vi "Dashboard Main.vi"() -> ()   [LabVIEW 2013]
uses:
  <vilib>/event_ctls.llb/eventvkey.ctl
  <vilib>/Rock Robotics/WPI/Dashboard/WPI_DashboardLogging Global.vi
  <vilib>/Utility/config.llb/Write Key (String).vi
  <vilib>/Utility/config.llb/Write Key (I32).vi
  <vilib>/Utility/config.llb/NI_LVConfig.lvlib
panel:
  out "Image Message":string="Timeout in Camera Communications"
  in  "Rec Mode":enum32{"Stop", "Record", "Playback"}(radio)
  in  "Dashboard Tab":T1(tab)
  out "RightJoystick":dbl(slide) scale=-1.0..1.0
  out "LeftJoystick":dbl(slide) scale=-1.0..1.0
  out "RightMotor":dbl(slide) scale=-1.0..1.0 scale format="%#.6g"
  out "StraightDrive":bool
  out "HalfDrive":bool
  in  "AccelRate":dbl(slide)=0.75 min=0.0 max=1.0 step=0.01 scale=0.0..1.0 scale format="%#_2g"
  out "LeftMotor":dbl(slide) scale=-1.0..1.0
  in  "Camera Settings":T2={"Frame Rate"=30, "Compression"=30, "Size"=1} {"Frame Rate" scale=1.0..30.0; "Size" items=["640x480", "320x240", "160x120"]}
  out "MotorSliders R":cluster{"MotorSlide1":dbl, "MotorSlide2":dbl} {"MotorSlide2" scale=-1.0..1.0 scale format="%#_2e"; "MotorSlide1" scale=-1.0..1.0 scale format="%#_2e"}
  out "MotorChart R":cluster{"Numeric":dbl, "Numeric":dbl}(graph)
  out "MotorSliders L":T3 {"MotorSlide4 2" scale=0.0..14.0 scale format="%#_2e"; "MotorSlide2" scale=-1.0..1.0 scale format="%#_2e"; "MotorSlide1" scale=-1.0..1.0 scale format="%#_2e"}
  out "MotorChart L":T4(graph)
  out "Mode":T5(ring)=enum."Auto Disabled"
  out "Camera IP":string
  in  "DB Camera Config":bool
  out "fps":dbl format="%#.1g"
  out "Mbps":dbl format="%#.1g"
  out "Mbps 2":bool
  out "LED 1":bool
  in  "Slider 1":dbl(slide) scale=0.0..100.0
  in  "Checkbox 2":bool
  in  "Checkbox 1":bool
  in  "Test Slider":dbl(slide) scale=0.0..100.0 scale format="%#_3g"
  in  "On/Off":bool caption="Solenoid"
  in  "Test Name":u16(ring) items=["Select the test to run...", "Example Test", "-------------------------------", "List of tests is built in robot code.", "Replace with your own automated tests."]
  in  "Test Tree":string(tree)
  in  "Motor":cluster{"Value":dbl, "Enable":bool} {"Value" scale=-1.0..1.0 scale format="%#_3g"}
  out "Progress":T6 {"Test Progress" scale=0.0..100.0}
  in  "Rev/Fwd":cluster{"Forward":bool, "Reverse":bool}
  in  "Test Ring":u16(ring) items=["Auto", "Fixed indoor", "Fixed outdoor 1", "Fixed outdoor 2", "Fixed fluorescent 1", "Fixed fluorescent 2", "Hold current"]
  in  "Listbox":i32(listbox)
  out "Tree":string(tree)
  out "Camera Image":T7(plugin-control)
  in  "Enable":bool
  # "Left"
  # "Front"
  # "Right"
  # "Battery"
  # "Customize by placing controls and indicators here and name to\nmatch Dashboard Variables on robot."
  # "This tab is a great place for autonomous settings and validation.\nCustomize by placing controls and indicators here and name to\nmatch Dashboard Variables on robot."
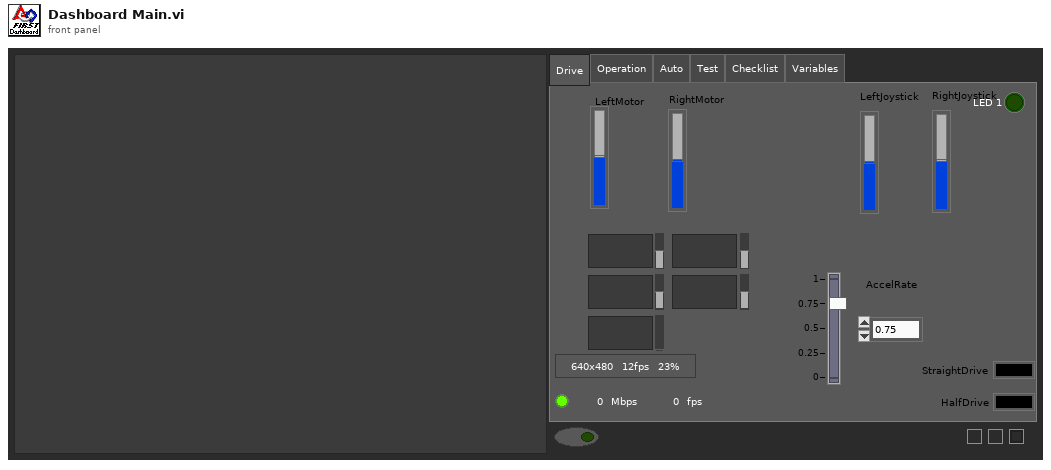
[diagram p1: front panel]
types:
  T1 = enum32{"Drive", "Operation", "Auto", "Test", "Checklist", "Variables"}
  T2 = cluster{"Frame Rate":i32, "Compression":i32, "Size":u16}
  T3 = cluster{"MotorSlide1":dbl, "MotorSlide2":dbl, "MotorSlide4 2":dbl}
  T4 = cluster{"Numeric":dbl, "Numeric":dbl, "Battery":sgl}
  T5 = enum8{"Tele-Op Disabled", "Tele-Op Enabled", "Auto Disabled", "Auto Enabled", "Test Disabled", "Test Enabled", ""}
  T6 = cluster{"Test Progress":u8, "Test Progress Text":string}
  T7 = typedef "IMAQ Image.ctl" = refnum<image>
  T8 = typedef "Image Type" = u32
  T9 = cluster{"Digital Inputs":bool[], "Digital Outputs":bool[]}
  T10 = cluster{"Competition mode":bool, "Robot Link":bool, "Autonomous":bool, "Enabled":bool, "E-Stop":bool, "Simulated":bool, "TestMode":bool, "Docked Window":bool}
  T11 = typedef "NI_LVConfig.lvlib/Config Data RefNum.ctl" = refnum<k1>
  T12 = typedef "eventvkey.ctl" = enum16{"ASCII", "Enter", "Return", "Shift", "Ctrl", "Alt", "Cmd", "Opt", "Caps", "NumLock", "Clear", "Break", "Up", "Down", "Left", "Right", "Insert", "Delete", "Home", "End", "PageUp", "PageDown", "Escape", "Help", "Pause", "ScrollLock", "F1", "F2", "F3", "F4", "F5", "F6", "F7", "F8", "F9", "F10", "F11", "F12", "F13", "F14", "F15", "F16", "F17", "F18", "F19", "F20", "F21", "F22", "F23", "F24", "Play", "VolumeUp", "VolumeDown", "Mute", "Two Byte Char"}
  T13 = cluster{"Image Size":bool, "Image Type":bool, "Pixel Value":bool, "ROI Information":bool, "Zoom Factor":bool}
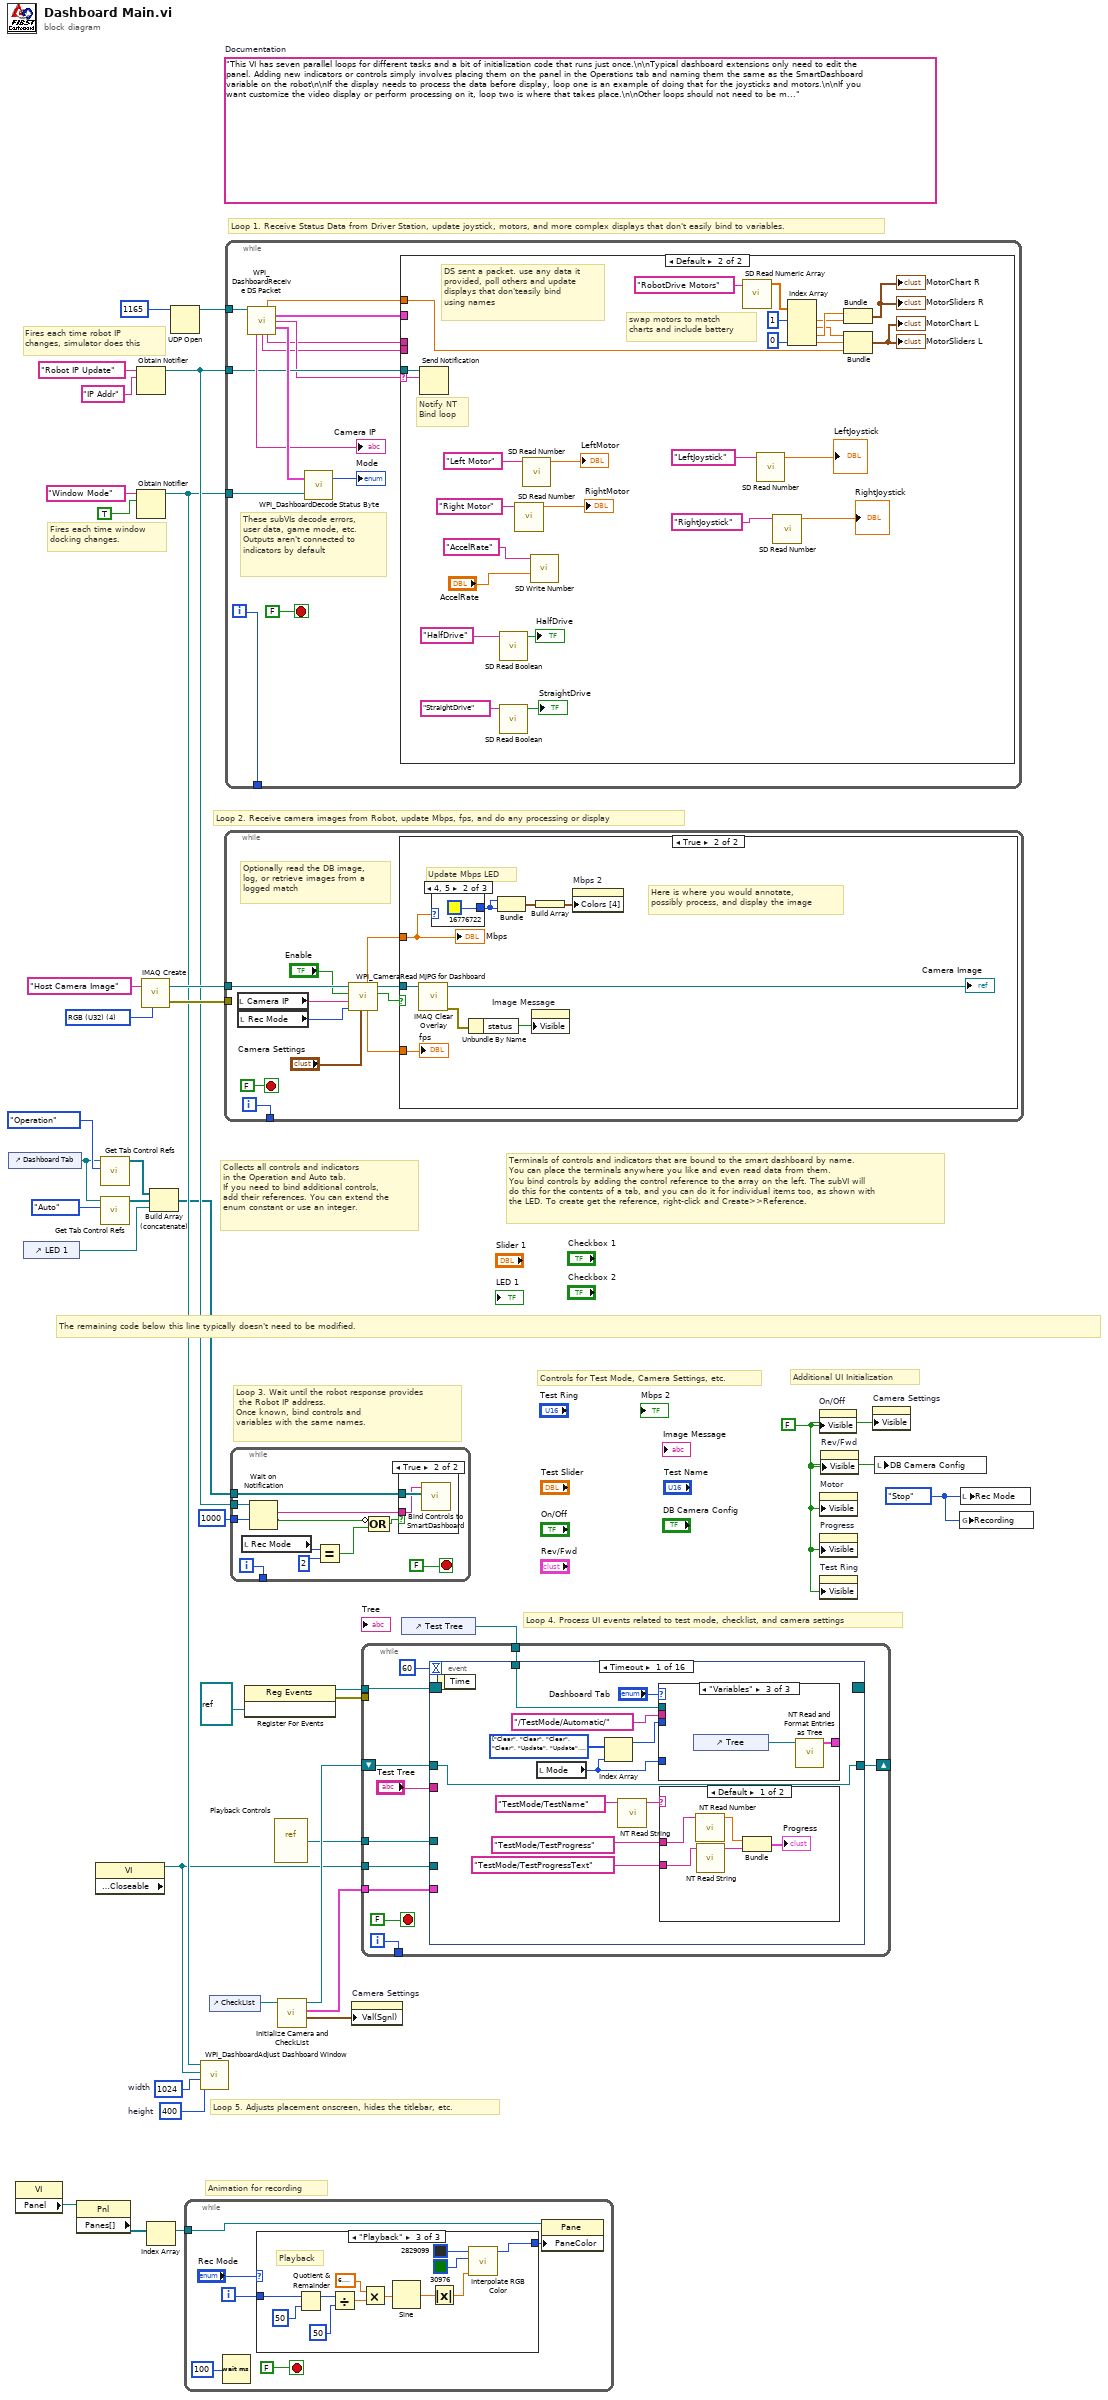
[diagram p0: block diagram]
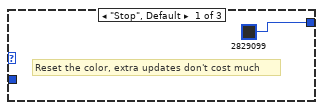
[diagram p2: hidden frame]
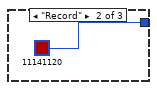
[diagram p3: hidden frame]
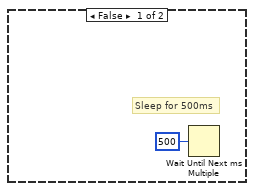
[diagram p5: hidden frame]
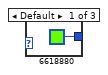
[diagram p6: hidden frame]
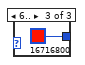
[diagram p7: hidden frame]
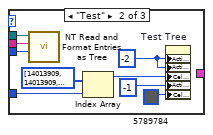
[diagram p9: hidden frame]
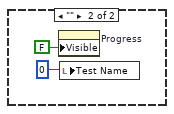
[diagram p10: hidden frame]
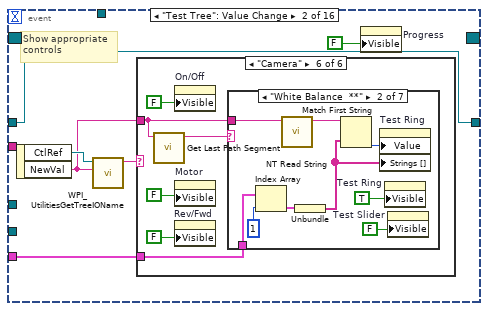
[diagram p11: hidden frame]
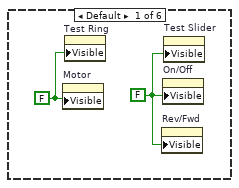
[diagram p12: hidden frame]
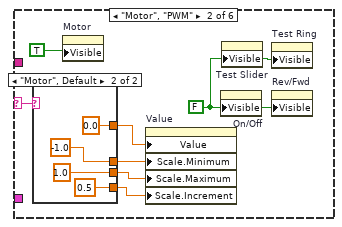
[diagram p13: hidden frame]
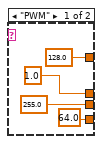
[diagram p14: hidden frame]
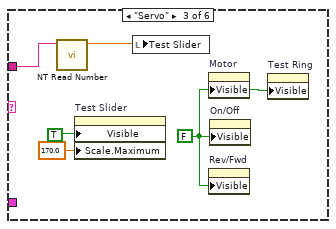
[diagram p15: hidden frame]
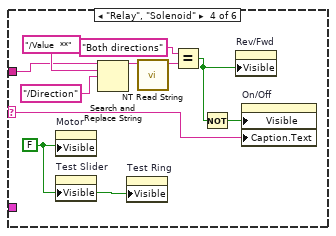
[diagram p16: hidden frame]
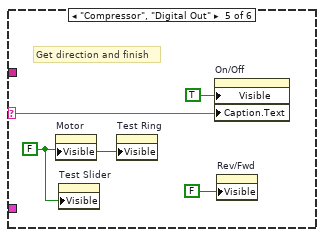
[diagram p17: hidden frame]
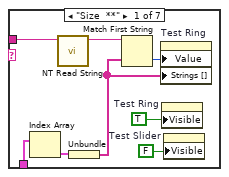
[diagram p18: hidden frame]
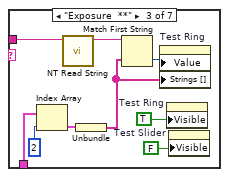
[diagram p19: hidden frame]
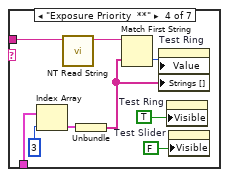
[diagram p20: hidden frame]
diagram:
  w8 = enum32{"Stop", "Record", "Playback"}."Stop" ("Rec Mode")
  w11 = 400  # height
  w12 = 1024  # width
  w25 = FALSE ("Visible")
  (unwired) "This VI has seven parallel loops for different tasks and a bit of initialization code that runs just once.\n\nTypical dashboard extensions only need to edit the panel. Adding new indicators or controls simply involves placing them on the panel in the Operations tab and naming them the same as the SmartDashboard variable on the robot\n\nIf the display needs to process the data before display, loop one is an example of doing that for the joysticks and motors.\n\nIf you want customize the video display or perform processing on it, loop two is where that takes place.\n\nOther loops should not need to be modified. They are pretty standard, and document the task they perform."  # Documentation
  w35 = T8 4 items=["Grayscale (U8)", "Grayscale (I16)", "Grayscale (SGL)", "Complex (CSG)", "RGB (U32)", "HSL (U32)", "RGB (U64)"] ("Image Type")
  # "Controls for Test Mode, Camera Settings, etc."
  # "Additional UI Initialization"
  # "Animation for recording"
  # "Fires each time robot IP\nchanges, simulator does this"
  # "Fires each time window\ndocking changes."
  # "Collects all controls and indicators\nin the Operation and Auto tab.\nIf you need to bind additional controls,\nadd their references. You can extend the\nenum constant or use an integer."
  # "The remaining code below this line typically doesn't need to be modified."
  # "Loop 4. Process UI events related to test mode, checklist, and camera settings"
  # "Terminals of controls and indicators that are bound to the smart dashboard by name.\nYou can place the terminals anywhere you like and even read data from them.\nYou bind controls by adding the control reference to the array on the left. The subVI will\ndo this for the contents of a tab, and you can do it for individual items too, as shown with\nthe LED. To create get the reference, right-click and Create>>Reference."
  # "Loop 3. Wait until the robot response provides\n the Robot IP address.\nOnce known, bind controls and\nvariables with the same names."
  # "Loop 5. Adjusts placement onscreen, hides the titlebar, etc."
  # "Loop 1. Receive Status Data from Driver Station, update joystick, motors, and more complex displays that don't easily bind to variables."
  # "Loop 2. Receive camera images from Robot, update Mbps, fps, and do any processing or display"
  n1 = control-ref of="Dashboard Tab"() -> (w6:refnum<vi>)
  n2 = property class="VI"() -> ("Panel"=w19:refnum<vi>)  [unwired: 2 in, 2 out]
  n3 = control-ref of="LED 1"() -> (w1:refnum<vi>)
  n4 = property class="Pnl"(reference=w19) -> ("Panes[]"=w20:refnum<vi>[])  [unwired: 1 in, 2 out]
  n5 = property class="VI" props=["Front Panel.Closeable"]() -> (reference out=w7:refnum<vi>)  [unwired: 2 in, 2 out]
  n6 = call <vilib>:"Get Tab Control Refs.vi"("Page Index"=T1."Operation" ("Dashboard Tab"), "TabControl in"=w6) -> ("ControlsOnPage"=w4:refnum<vi>[])  [unwired: 9 in]
  n7 = call <vilib>:"Get Tab Control Refs.vi"("Page Index"=T1."Auto" ("Dashboard Tab"), "TabControl in"=w6) -> ("ControlsOnPage"=w5:refnum<vi>[])  [unwired: 9 in]
  n8 = Obtain Notifier(name (unnamed)="Robot IP Update", notification data type="IP Addr" ("name (unnamed)")) -> (notifier out=w29:refnum<notifier>)  [unwired: 2 in, 2 out]
  n9 = Obtain Notifier(name (unnamed)="Window Mode", notification data type=TRUE) -> (notifier out=w10:refnum<notifier>)  [unwired: 2 in, 2 out]
  n10 = call "IMAQ Create"("Image Name"="Host Camera Image", "Image Type"=w35) -> ("New Image"=w33:T7, "error out"=w32:errorcluster)  [unwired: 2 in, 1 out]
  n11 = Index Array(array=w20) -> (element=w18:refnum<vi>)  [unwired: 1 in]
  n12 = Build Array (concatenate)(w4, w5, w1) -> (w3:refnum<vi>[])
  n13 = UDP Open(11:u16 1165 ("port")) -> (port=w36:refnum<k16>)  [unwired: 2 in, 4 out]
  n14 = while {
    tunnel: w18 -> [w39]
    i -> [w42]
    stop <- FALSE stop-if-true
    n15 = Wait (ms)(milliseconds to wait=u32 100) -> ()  [unwired: 1 out]
    n16 = case shown="\"Playback\"" "Rec Mode" {
      tunnel: w42 -> [_ _ w57]
      tunnel: [u32 2829099 ("Base Color") u32 11141120 ("Target Color") w46] -> w38
      frame "Stop", Default {
        # "Reset the color, extra updates don't cost much"
      }
      frame "Record" {
      }
      frame "Playback" {
        # "Playback"
        n17 = Quotient & Remainder(x=w57, y=u32 50 ("milliseconds to wait")) -> (x-y*floor(x/y)=w53:u32)  [unwired: 1 out]
        n18 = Divide(x=w53, y=u32 50 ("milliseconds to wait")) -> (x/y=w50:dbl)
        n19 = Multiply(x=6.283185307179586, y=w50) -> (x*y=w55:dbl)
        n20 = Sine(x=w55) -> (sin(x)=w54:dbl)
        n21 = Absolute Value(x=w54) -> (abs(x)=w47:dbl)
        n22 = call "Interpolate RGB Color.vi"("Proportion"=w47, "Target Color"=u32 30976, "Base Color"=u32 2829099) -> ("Result Color"=w46:u32)  [unwired: 8 in]
      }
    }
    n23 = property class="Pane"(reference=w39, "PaneColor"=w38) -> ()  [unwired: 1 in, 2 out]
  }
  n24 = call <vilib>:"WPI_DashboardAdjust Dashboard Window.vi"("height"=w11, "width"=w12, "reference in"=w7, "Notifier in"=w10) -> ()  [unwired: 8 in]
  n25 = control-ref of="CheckList"() -> (w9:refnum<vi>)
  n26 = while {
    tunnel: w33 -> [w66]
    tunnel: w32 -> [_]
    tunnel: [w67] -> _
    i -> [w67]
    stop <- FALSE stop-if-true
    # "Optionally read the DB image,\nlog, or retrieve images from a\nlogged match"
    n27 = local read "Camera IP"() -> (w59:string)
    n28 = local read "Rec Mode"() -> (w58:enum32{"Stop", "Record", "Playback"})
    n29 = call <vilib>:"WPI_CameraRead MJPG for Dashboard.vi"("Camera Settings"="Camera Settings", "Rec Mode"=w58, "Camera IP"=w59, "Enable"="Enable", "Refnum in"=w66) -> ("Active"=w63:bool, "Refnum out"=w65:T7, "FPS"=w62:dbl, "Bandwidth (Mbps)"=w61:dbl)  [unwired: 3 in]
    n30 = case shown="True" w63 {
      tunnel: w65 -> [_ w73]
      tunnel: w61 -> [_ w72]
      tunnel: w62 -> [_ w70]
      frame False {
        # "Sleep for 500ms"
        n31 = Wait Until Next ms Multiple(millisecond multiple=u32 500) -> ()  [unwired: 1 out]
      }
      frame True {
        # "Here is where you would annotate,\npossibly process, and display the image"
        # "Update Mbps LED"
        n32 = call "IMAQ Clear Overlay"("Image"=w73) -> ("error out"=w77:errorcluster, "Image Out"=→"Camera Image":T7)  [unwired: 2 in, 7 out]
        n33 = case shown="4, 5" w72 {
          tunnel: [u32 6618880 ("Color Box") u32 16776722 ("Color Box") u32 16716800 ("Color Box")] -> w74
          frame Default {
          }
          frame 4, 5 {
          }
          frame 6.. {
          }
        }
        n34 = Unbundle By Name(w77) -> ("status"=w78:bool)
        n35 = Bundle("Color Box"=w74, "Color Box"=w74) -> (w76:cluster{"Color Box":u32, "Color Box":u32})  [unwired: 1 out]
        n36 = property on="Image Message" class="Str"("Visible"=w78) -> ()  [unwired: 2 in, 2 out]
        n37 = Build Array(w76) -> (w75:cluster{"Color Box":u32, "Color Box":u32}[])
        n38 = property on="Mbps 2" class="Bool (strict)"("Colors [4]"=w75) -> ()  [unwired: 2 in, 2 out]
        "Mbps" <- w72
        "fps" <- w70
      }
    }
  }
  n39 = while {
    tunnel: w36 -> [w92]
    tunnel: w29 -> [w87]
    tunnel: w10 -> [w91]
    tunnel: [w88] -> _
    i -> [w88]
    stop <- FALSE stop-if-true
    # "These subVIs decode errors, user data, game mode, etc.\nOutputs aren't connected to indicators by default"
    n40 = call <vilib>:"WPI_DashboardReceive DS Packet.vi"("Recv Socket"=w92) -> ("Battery"=w82:sgl, "Driver Station"=w83:T9, "Robot IP Address"=w86:string, "Status"=w93:T10, "Camera IP Address"=→"Camera IP":string, "Low Priority User Data"=w85:string, "High Priority User Data"=w84:string)  [unwired: 1 in, 7 out]
    n41 = call <vilib>:"WPI_DashboardDecode Status Byte.vi"("Window Mode Notifier"=w91, "Status"=w93) -> ("Mode"=→"Mode":T5)  [unwired: 1 out]
    n42 = case shown="Default" w86 {
      selector: w86 -> [_ w119]
      tunnel: w87 -> [_ w120]
      tunnel: w85 -> [_ _]
      tunnel: w84 -> [_ _]
      tunnel: w83 -> [_ _]
      tunnel: w82 -> [_ w118]
      frame "0.0.0.0" {
        # "DS not sending packets, or no robot exists yet.\nDon't poll the variables"
      }
      frame Default {
        # "Notify NT\nBind loop"
        # "DS sent a packet. use any data it\nprovided, poll others and update\ndisplays that don'teasily bind\nusing names"
        # "swap motors to match\ncharts and include battery"
        n43 = Send Notification(notification=w119, notifier=w120) -> ()  [unwired: 1 in, 2 out]
        n44 = call <vilib>:"SD Read Boolean.vi"("Name"="HalfDrive") -> ("Boolean"=→"HalfDrive":bool)  [unwired: 8 in, 2 out]
        n45 = call <vilib>:"SD Read Boolean.vi"("Name"="StraightDrive") -> ("Boolean"=→"StraightDrive":bool)  [unwired: 8 in, 2 out]
        n46 = call <vilib>:"SD Read Number.vi"("Name"="Right Motor") -> ("Numeric"=→"RightMotor":dbl)  [unwired: 8 in, 2 out]
        n47 = call <vilib>:"SD Read Number.vi"("Name"="Left Motor") -> ("Numeric"=→"LeftMotor":dbl)  [unwired: 8 in, 2 out]
        n48 = call <vilib>:"SD Write Number.vi"("Numeric"="AccelRate", "Name"="AccelRate") -> ()  [unwired: 8 in, 2 out]
        n49 = call <vilib>:"SD Read Numeric Array.vi"("Name"="RobotDrive Motors") -> ("Numeric Array"=w117:dbl[])  [unwired: 8 in, 2 out]
        n50 = call <vilib>:"SD Read Number.vi"("Name"="LeftJoystick") -> ("Numeric"=→"LeftJoystick":dbl)  [unwired: 8 in, 2 out]
        n51 = call <vilib>:"SD Read Number.vi"("Name"="RightJoystick") -> ("Numeric"=→"RightJoystick":dbl)  [unwired: 8 in, 2 out]
        n52 = Index Array(array=w117, index #1=1, index #4=0) -> (element #1=w113:dbl, element #2=w112:dbl, element #3=w114:dbl, element #4=w109:dbl)  [unwired: 2 in]
        n53 = Bundle("Numeric"=w114, "Numeric"=w113) -> (→"MotorChart R" →"MotorSliders R":cluster{"Numeric":dbl, "Numeric":dbl})  [unwired: 1 in]
        n54 = Bundle("Numeric"=w112, "Numeric"=w109, "Battery"=w118) -> (→"MotorChart L" →"MotorSliders L":T4)  [unwired: 1 in]
      }
    }
  }
  n55 = while {
    tunnel: w3 -> [w132]
    tunnel: w29 -> [w130]
    tunnel: [w128] -> _
    tunnel: u32 1000 ("milliseconds to wait") -> [w127]
    i -> [w128]
    stop <- FALSE stop-if-true
    n56 = local read "Rec Mode"() -> (w123:enum32{"Stop", "Record", "Playback"})
    n57 = Wait on Notification(notifier=w130, timeout in ms (-1)=w127) -> (notification=w129:string, timed out?=w125:bool)  [unwired: 2 in, 2 out]
    n58 = Equal?(x=w123, y=u16 2 ("Rec Mode")) -> (x = y?=w124:bool)
    n59 = Compound Arithmetic op=OR(invert w125, w124) -> (w126:bool)
    n60 = case shown="True" w126 {
      tunnel: w132 -> [_ w134]
      tunnel: w129 -> [_ w133]
      frame False {
      }
      frame True {
        n61 = call <vilib>:"Bind Controls to SmartDashboard.vi"("Bound Control Refs"=w134, "Server IP Address"=w133) -> ()  [unwired: 10 in]
      }
    }
  }
  n62 = register-events(refnum<vi> refnum) -> (reference out=w16:refnum<event-registration>, error out=w15:errorcluster)  [unwired: 2 in]
  n63 = vi-ref "Playback Controls.vi"() -> (w17:refnum<vi>)
  n64 = call "Initialize Camera and CheckList.vi"("ListBox in"=w9) -> ("Cluster"=w23:cluster{"value":i32, "value":i32, "index":i32}, "Array"=w24:cluster{string[]}[], "File Refnum"=w22:T11)  [unwired: 8 in]
  n65 = property on="Camera Settings" class="Clust (strict)"("Val(Sgnl)"=w23) -> ()  [unwired: 2 in, 2 out]
  n66 = control-ref of="Test Tree"() -> (w21:refnum<vi>)
  n67 = while {
    tunnel: w24 -> [w142]
    shift-right: [w141] -> _
    shift-left: w22 -> [w140]
    tunnel: [w139] -> _
    tunnel: w21 -> [w138]
    tunnel: w17 -> [w137]
    tunnel: w16 -> [w136]
    tunnel: w15 -> [_]
    tunnel: w7 -> [w135]
    i -> [w139]
    stop <- FALSE stop-if-true
    n68 = event shown="[0] Timeout" {
      selector: w136 -> [_ _ _ _ _ _ _ _ _ _ _ _ _ _ _ _]
      dyn-events: [_ _ _ _ _ _ _ _ _ _ _ _ _ w380 _ _] -> _
      timeout: u32 60 ("milliseconds to wait") -> [_ _ _ _ _ _ _ _ _ _ _ _ _ _ _ _]
      tunnel: w138 -> [w152 _ _ _ _ _ _ _ _ _ _ _ _ _ _ _]
      tunnel: "Test Tree" -> [_ _ _ _ _ _ _ _ w349 w357 w359 w363 w371 _ _ _]
      tunnel: w142 -> [_ w176 _ _ _ _ w313 w343 _ _ _ _ _ _ _ _]
      tunnel: [w146 w175 w274 w279 w287 w299 w312 w336 w348 w355 w358 w362 w370 w382 w396 w397] -> w141
      tunnel: w140 -> [w146 w175 w274 w279 w287 w299 w311 w336 w348 w355 w358 w362 w370 w382 w396 w397]
      tunnel: w137 -> [_ _ _ _ _ _ _ _ _ _ _ _ _ w383 _ w400]
      tunnel: w135 -> [_ _ _ _ _ _ _ _ _ _ _ _ _ w378 _ _]
      event Timeout {
        w151 = enum16{"Update", "Clear"}[] [enum."Clear", enum."Clear", enum."Clear", enum."Clear", enum."Update", enum."Update", enum."Clear"] items=["Update", "Clear"]
        n69 = event-data() -> ()  [unwired: 1 in, 1 out]
        n70 = local read "Mode"() -> (w149:T5)
        n71 = Index Array(array=w151, index=w149) -> (element=w150:enum16{"Update", "Clear"})
        n72 = call <vilib>:"NT Read String.vi"("Name"="TestMode/TestName") -> ("String"=w155:string)  [unwired: 9 in, 1 out]
        n73 = case shown="\"Variables\"" "Dashboard Tab" {
          tunnel: w152 -> [_ w165 _]
          tunnel: "/TestMode/Automatic/" ("Name Pattern") -> [_ w164 _]
          tunnel: w150 -> [_ w163 _]
          tunnel: w149 -> [_ w161 _]
          tunnel: [_ _ w167] -> _
          frame "Operation", Default {
          }
          frame "Test" {
            w160 = -2 ("Active Item:Row Number")
            n74 = call <vilib>:"NT Read and Format Entries as Tree.vi"("Operation"=w163, "Name Pattern"=w164, "Tree Refnum"=w165) -> ()  [unwired: 7 in, 2 out]
            n75 = Index Array(array=u32[] [14013909, 14013909, 14013909, 14013909, 14013909, 16777215, 14013909], index=w161) -> (element=w159:u32)
            n76 = property on="Test Tree" class="Tree (strict)"("Active Item Row Number"=w160, "ActiveColNum"=w160, "CellBG"=w159, "Active Item Row Number"=-1 ("Active Item:Row Number"), "CellBG"=u32 5789784 ("Color Box")) -> ()  [unwired: 2 in, 2 out]
          }
          frame "Variables" {
            n77 = control-ref of="Tree"() -> (w166:refnum<vi>)
            n78 = call <vilib>:"NT Read and Format Entries as Tree.vi"("Tree Refnum"=w166) -> ("Formatted Strings"=w167:cluster{"Name":string, "Value":string}[])  [unwired: 9 in, 1 out]
          }
        }
        n79 = case shown="Default" w155 {
          tunnel: "TestMode/TestProgress" ("Name") -> [w169 _]
          tunnel: "TestMode/TestProgressText" ("Name") -> [w168 _]
          frame Default {
            n80 = call <vilib>:"NT Read Number.vi"("Name"=w169) -> ("Numeric"=w170:dbl)  [unwired: 9 in, 1 out]
            n81 = call <vilib>:"NT Read String.vi"("Name"=w168) -> ("String"=w171:string)  [unwired: 9 in, 1 out]
            n82 = Bundle("Numeric"=w170, "String"=w171) -> (→"Progress":cluster{"Numeric":dbl, "String":string})  [unwired: 1 in]
          }
          frame "" {
            n83 = property on="Progress" class="Clust (strict)"("Visible"=FALSE) -> ()  [unwired: 2 in, 2 out]
            n84 = local write "Test Name"(u16 0) -> ()
          }
        }
      }
      event "Test Tree": Value Change {
        # "Show appropriate\ncontrols"
        n85 = event-data() -> ("CtlRef"=w179:refnum<vi>, "NewVal"=w177:string)  [unwired: 1 in]
        n86 = call <vilib>:"WPI_UtilitiesGetTreeIOName.vi"("NewVal"=w177, "TreeControl in"=w179) -> ("I/O Name"=w180:string)  [unwired: 9 in]
        n87 = case shown="\"Camera\"" w180 {
          selector: w180 -> [_ w187 _ w205 w214 _]
          tunnel: w177 -> [_ _ w202 w204 _ w221]
          tunnel: w176 -> [_ _ _ _ _ w220]
          frame Default {
            w182 = FALSE ("Visible")
            w181 = FALSE ("Visible")
            n88 = property on="Motor" class="Clust (strict)"("Visible"=w181) -> ()  [unwired: 2 in, 2 out]
            n89 = property on="Test Ring" class="Ring (strict)"("Visible"=w181) -> ()  [unwired: 2 in, 2 out]
            n90 = property on="Rev/Fwd" class="Clust (strict)"("Visible"=w182) -> ()  [unwired: 2 in, 2 out]
            n91 = property on="On/Off" class="Bool (strict)"("Visible"=w182) -> ()  [unwired: 2 in, 2 out]
            n92 = property on="Test Slider" class="Slide (strict)"("Visible"=w182) -> ()  [unwired: 2 in, 2 out]
          }
          frame "Motor", "PWM" {
            w188 = FALSE ("Visible")
            n93 = case shown="\"Motor\", Default" w187 {
              tunnel: [1.0 ("Value") -1.0 ("Value")] -> w186
              tunnel: [255.0 ("Value") 1.0 ("Value")] -> w185
              tunnel: [128.0 ("Value") 0.0 ("Value")] -> w184
              tunnel: [64.0 ("Value") 0.5 ("Value")] -> w183
              frame "PWM" {
              }
              frame "Motor", Default {
              }
            }
            n94 = property on="Motor" class="Clust (strict)"("Visible"=TRUE) -> ()  [unwired: 2 in, 2 out]
            n95 = property on="Value" class="Slide (strict)"("Value"=w184, "Scale.Minimum"=w186, "Scale.Maximum"=w185, "Scale.Increment"=w183) -> ()  [unwired: 2 in, 2 out]
            n96 = property on="On/Off" class="Bool (strict)"("Visible"=w188) -> ()  [unwired: 2 in, 2 out]
            n97 = property on="Test Slider" class="Slide (strict)"("Visible"=w188) -> ()  [unwired: 2 in, 2 out]
            n98 = property on="Test Ring" class="Ring (strict)"("Visible"=w188) -> ()  [unwired: 2 in, 2 out]
            n99 = property on="Rev/Fwd" class="Clust (strict)"("Visible"=w188) -> ()  [unwired: 2 in, 2 out]
          }
          frame "Servo" {
            w200 = FALSE ("Visible")
            n100 = call <vilib>:"NT Read Number.vi"("Name"=w202) -> ("Numeric"=w201:dbl)  [unwired: 9 in, 1 out]
            n101 = property on="Test Slider" class="Slide (strict)"("Visible"=TRUE, "Scale.Maximum"=170.0 ("Scale.Range:Maximum")) -> ()  [unwired: 2 in, 2 out]
            n102 = local write "Test Slider"(w201) -> ()
            n103 = property on="Motor" class="Clust (strict)"("Visible"=w200) -> ()  [unwired: 2 in, 2 out]
            n104 = property on="Rev/Fwd" class="Clust (strict)"("Visible"=w200) -> ()  [unwired: 2 in, 2 out]
            n105 = property on="On/Off" class="Bool (strict)"("Visible"=w200) -> ()  [unwired: 2 in, 2 out]
            n106 = property on="Test Ring" class="Ring (strict)"("Visible"=w200) -> ()  [unwired: 2 in, 2 out]
          }
          frame "Relay", "Solenoid" {
            w203 = FALSE ("Visible")
            n107 = property on="Motor" class="Clust (strict)"("Visible"=w203) -> ()  [unwired: 2 in, 2 out]
            n108 = property on="Test Slider" class="Slide (strict)"("Visible"=w203) -> ()  [unwired: 2 in, 2 out]
            n109 = Search and Replace String(input string=w204, search string="/Value  **", replace string="/Direction") -> (result string=w210:string)  [unwired: 5 in, 3 out]
            n110 = property on="Test Ring" class="Ring (strict)"("Visible"=w203) -> ()  [unwired: 2 in, 2 out]
            n111 = call <vilib>:"NT Read String.vi"("Name"=w210) -> ("String"=w208:string)  [unwired: 9 in, 1 out]
            n112 = Equal?(x="Both directions", y=w208) -> (x = y?=w206:bool)
            n113 = Not(x=w206) -> (.not. x?=w207:bool)
            n114 = property on="Rev/Fwd" class="Clust (strict)"("Visible"=w206) -> ()  [unwired: 2 in, 2 out]
            n115 = property on="On/Off" class="Bool (strict)"("Visible"=w207, "Caption.Text"=w205) -> ()  [unwired: 2 in, 2 out]
          }
          frame "Compressor", "Digital Out" {
            w213 = FALSE ("Visible")
            # "Get direction and finish"
            n116 = property on="Motor" class="Clust (strict)"("Visible"=w213) -> ()  [unwired: 2 in, 2 out]
            n117 = property on="Test Slider" class="Slide (strict)"("Visible"=w213) -> ()  [unwired: 2 in, 2 out]
            n118 = property on="Test Ring" class="Ring (strict)"("Visible"=w213) -> ()  [unwired: 2 in, 2 out]
            n119 = property on="On/Off" class="Bool (strict)"("Visible"=TRUE, "Caption.Text"=w214) -> ()  [unwired: 2 in, 2 out]
            n120 = property on="Rev/Fwd" class="Clust (strict)"("Visible"=FALSE) -> ()  [unwired: 2 in, 2 out]
          }
          frame "Camera" {
            n121 = call <vilib>:"Get Last Path Segment.vi"("String in"=w221) -> ("String out"=w222:string)  [unwired: 10 in]
            n122 = property on="On/Off" class="Bool (strict)"("Visible"=FALSE) -> ()  [unwired: 2 in, 2 out]
            n123 = property on="Motor" class="Clust (strict)"("Visible"=FALSE) -> ()  [unwired: 2 in, 2 out]
            n124 = property on="Rev/Fwd" class="Clust (strict)"("Visible"=FALSE) -> ()  [unwired: 2 in, 2 out]
            n125 = case shown="\"White Balance  **\"" w222 {
              tunnel: w221 -> [w228 w237 w246 w255 w264 _ w270]
              tunnel: w220 -> [w226 w234 w243 w252 w261 _ _]
              frame "Size  **" {
                n126 = Index Array(array=w226) -> (element=w225:cluster{string[]})  [unwired: 1 in]
                n127 = call <vilib>:"NT Read String.vi"("Name"=w228) -> ("String"=w227:string)  [unwired: 9 in, 1 out]
                n128 = Unbundle(w225) -> (w223:string[])
                n129 = Match First String(2:w223, 3:w227) -> (0:w224:i32)  [unwired: 1 out]
                n130 = property on="Test Ring" class="Ring (strict)"("Value"=w224, "Strings []"=w223) -> ()  [unwired: 2 in, 2 out]
                n131 = property on="Test Ring" class="Ring (strict)"("Visible"=TRUE) -> ()  [unwired: 2 in, 2 out]
                n132 = property on="Test Slider" class="Slide (strict)"("Visible"=FALSE) -> ()  [unwired: 2 in, 2 out]
              }
              frame "White Balance  **" {
                n133 = Index Array(array=w234, index=1) -> (element=w235:cluster{string[]})
                n134 = call <vilib>:"NT Read String.vi"("Name"=w237) -> ("String"=w236:string)  [unwired: 9 in, 1 out]
                n135 = Unbundle(w235) -> (w232:string[])
                n136 = Match First String(2:w232, 3:w236) -> (0:w231:i32)  [unwired: 1 out]
                n137 = property on="Test Ring" class="Ring (strict)"("Value"=w231, "Strings []"=w232) -> ()  [unwired: 2 in, 2 out]
                n138 = property on="Test Ring" class="Ring (strict)"("Visible"=TRUE) -> ()  [unwired: 2 in, 2 out]
                n139 = property on="Test Slider" class="Slide (strict)"("Visible"=FALSE) -> ()  [unwired: 2 in, 2 out]
              }
              frame "Exposure  **" {
                n140 = Index Array(array=w243, index=2) -> (element=w244:cluster{string[]})
                n141 = call <vilib>:"NT Read String.vi"("Name"=w246) -> ("String"=w245:string)  [unwired: 9 in, 1 out]
                n142 = Unbundle(w244) -> (w240:string[])
                n143 = Match First String(2:w240, 3:w245) -> (0:w241:i32)  [unwired: 1 out]
                n144 = property on="Test Ring" class="Ring (strict)"("Value"=w241, "Strings []"=w240) -> ()  [unwired: 2 in, 2 out]
                n145 = property on="Test Ring" class="Ring (strict)"("Visible"=TRUE) -> ()  [unwired: 2 in, 2 out]
                n146 = property on="Test Slider" class="Slide (strict)"("Visible"=FALSE) -> ()  [unwired: 2 in, 2 out]
              }
              frame "Exposure Priority  **" {
                n147 = Index Array(array=w252, index=3) -> (element=w253:cluster{string[]})
                n148 = call <vilib>:"NT Read String.vi"("Name"=w255) -> ("String"=w254:string)  [unwired: 9 in, 1 out]
                n149 = Unbundle(w253) -> (w249:string[])
                n150 = Match First String(2:w249, 3:w254) -> (0:w250:i32)  [unwired: 1 out]
                n151 = property on="Test Ring" class="Ring (strict)"("Value"=w250, "Strings []"=w249) -> ()  [unwired: 2 in, 2 out]
                n152 = property on="Test Ring" class="Ring (strict)"("Visible"=TRUE) -> ()  [unwired: 2 in, 2 out]
                n153 = property on="Test Slider" class="Slide (strict)"("Visible"=FALSE) -> ()  [unwired: 2 in, 2 out]
              }
              frame "Color Enable  **" {
                n154 = Index Array(array=w261, index=4) -> (element=w262:cluster{string[]})
                n155 = call <vilib>:"NT Read String.vi"("Name"=w264) -> ("String"=w263:string)  [unwired: 9 in, 1 out]
                n156 = Unbundle(w262) -> (w258:string[])
                n157 = Match First String(2:w258, 3:w263) -> (0:w259:i32)  [unwired: 1 out]
                n158 = property on="Test Ring" class="Ring (strict)"("Value"=w259, "Strings []"=w258) -> ()  [unwired: 2 in, 2 out]
                n159 = property on="Test Ring" class="Ring (strict)"("Visible"=TRUE) -> ()  [unwired: 2 in, 2 out]
                n160 = property on="Test Slider" class="Slide (strict)"("Visible"=FALSE) -> ()  [unwired: 2 in, 2 out]
              }
              frame Default {
                n161 = property on="Test Ring" class="Ring (strict)"("Visible"=FALSE) -> ()  [unwired: 2 in, 2 out]
                n162 = property on="Test Slider" class="Slide (strict)"("Visible"=FALSE) -> ()  [unwired: 2 in, 2 out]
              }
              frame "Brightness  **", "Color Level  **", "Compression  **", "FPS  **", "Sharpness  **" {
                n163 = call <vilib>:"NT Read Number.vi"("Name"=w270) -> ("Numeric"=w269:dbl)  [unwired: 9 in, 1 out]
                n164 = local write "Test Slider"(w269) -> ()
                n165 = property on="Test Slider" class="Slide (strict)"("Visible"=TRUE, "Scale.Maximum"=100.0 ("Scale.Range:Maximum")) -> ()  [unwired: 2 in, 2 out]
                n166 = property on="Test Ring" class="Ring (strict)"("Visible"=FALSE) -> ()  [unwired: 2 in, 2 out]
              }
            }
          }
        }
        n167 = property on="Progress" class="Clust (strict)"("Visible"=FALSE) -> ()  [unwired: 2 in, 2 out]
      }
      event "Test Name": Mouse Enter {
        # "Populate the ring with the list of tests"
        n168 = event-data() -> ()  [unwired: 1 in, 1 out]
        n169 = call <vilib>:"NT Read String Array.vi"("Name"="TestMode/TestList") -> ("String Array"=w278:string[])  [unwired: 9 in, 1 out]
        n170 = Build Array (concatenate)("Select the test to run...", w278) -> (w277:string[])
        n171 = property on="Test Name" class="Ring (strict)"("Strings []"=w277) -> ()  [unwired: 2 in, 2 out]
      }
      event "Test Name": Value Change {
        w280 = FALSE ("Visible")
        # "Tell the robot the test name to run"
        n172 = event-data() -> ("NewVal"=w284:u16)  [unwired: 1 in]
        n173 = property on="Test Name" class="Ring (strict)"() -> ("Strings []"=w285:string[])  [unwired: 2 in, 2 out]
        n174 = local write "Progress"(T6 {"Test Progress"=0, "Test Progress Text"=""} ("Progress")) -> ()
        n175 = Index Array(array=w285, index=w284) -> (element=w283:string)
        n176 = call <vilib>:"NT Write String.vi"("String"=w283, "Name"="TestMode/TestName") -> ()  [unwired: 9 in, 1 out]
        n177 = property on="Progress" class="Clust (strict)"("Visible"=TRUE) -> ()  [unwired: 2 in, 2 out]
        n178 = property on="Motor" class="Clust (strict)"("Visible"=w280) -> ()  [unwired: 2 in, 2 out]
        n179 = property on="Test Slider" class="Slide (strict)"("Visible"=w280) -> ()  [unwired: 2 in, 2 out]
        n180 = property on="On/Off" class="Bool (strict)"("Visible"=w280) -> ()  [unwired: 2 in, 2 out]
        n181 = property on="Rev/Fwd" class="Clust (strict)"("Visible"=w280) -> ()  [unwired: 2 in, 2 out]
        n182 = property on="Test Ring" class="Ring (strict)"("Visible"=w280) -> ()  [unwired: 2 in, 2 out]
      }
      event "Listbox": Double Click {
        n183 = event-data() -> ("PlatMods.Shift"=w288:bool, "Row"=w290:i32)  [unwired: 1 in]
        n184 = case shown="True" w288 {
          tunnel: w290 -> [w294 _]
          tunnel: 1 -> [w293 _]
          frame False {
            n185 = property on="Listbox" class="LstBox (strict)"() -> ("Item Symbols"=w292:i32[])  [unwired: 2 in, 2 out]
            n186 = Replace Array Subset(array=w292, new element=w293, index=w294) -> (w291:i32[])
            n187 = property on="Listbox" class="LstBox (strict)"("Item Symbols"=w291) -> ()  [unwired: 2 in, 2 out]
          }
          frame True {
            w295 = 0 ("Top Row")
            n188 = property on="Listbox" class="LstBox (strict)"() -> ("Number of Rows"=w297:u32)  [unwired: 2 in, 2 out]
            n189 = Initialize Array(0, w297) -> (w296:i32[])
            n190 = property on="Listbox" class="LstBox (strict)"("Top Row"=w295, "Value"=w295, "Item Symbols"=w296) -> ()  [unwired: 2 in, 2 out]
          }
        }
      }
      event "Listbox": Key Down {
        n191 = event-data() -> ("VKey"=w301:T12)  [unwired: 1 in]
        n192 = case shown="\"Left\", \"Right\"" w301 {
          selector: w301 -> [w306 _]
          tunnel: eventvkey."Left" ("VKey") -> [w304 _]
          frame "Left", "Right" {
            n193 = Equal?(x=w304, y=w306) -> (x = y?=w305:bool)
            n194 = Select(t=0, s=w305, f=1) -> (s? t:f=w307:i32)
            n195 = property on="Listbox" class="LstBox (strict)"() -> ("Item Symbols"=w310:i32[])  [unwired: 2 in, 2 out]
            n196 = Replace Array Subset(array=w310, new element=w307, index="Listbox") -> (w309:i32[])
            n197 = property on="Listbox" class="LstBox (strict)"("Item Symbols"=w309) -> ()  [unwired: 2 in, 2 out]
          }
          frame Default {
          }
        }
      }
      event "DB Camera Config": Value Change {
        n198 = event-data() -> ("NewVal"=w314:bool)  [unwired: 1 in]
        n199 = case shown="False" w314 {
          tunnel: w313 -> [w323 _]
          tunnel: [w316 w334] -> w312
          tunnel: w311 -> [w315 w334]
          frame False {
            w330 = "Camera"
            w333 = FALSE ("Visible")
            n200 = local read "Camera Settings"() -> (w322:T2)
            n201 = Index Array(array=w323) -> (element=w326:cluster{string[]})  [unwired: 1 in]
            n202 = Unbundle(w322) -> ("Frame Rate"=w321:i32, "Compression"=w320:i32, "Size"=w324:u16)
            n203 = Unbundle(w326) -> (w325:string[])
            n204 = Index Array(array=w325, index=w324) -> (element=w319:string)
            n205 = call-poly <vilib>:"Write Key.vi"("section"=w330, "value"=w319, "key"="Size", "refnum"=w315) -> ("refnum out"=w332:T11)  [unwired: 2 in, 5 out]
            n206 = call-poly <vilib>:"Write Key.vi"("section"=w330, "value"=w321, "key"="FrameRate", "refnum"=w332) -> ("refnum out"=w331:T11)  [unwired: 1 in, 6 out]
            n207 = property on="Camera Settings" class="Clust (strict)"("Visible"=w333) -> ()  [unwired: 2 in, 2 out]
            n208 = local write "DB Camera Config"(w333) -> ()
            n209 = call-poly <vilib>:"Write Key.vi"("section"=w330, "value"=w320, "key"="Compression", "refnum"=w331) -> ("refnum out"=w317:T11)  [unwired: 1 in, 6 out]
            n210 = call <vilib>:"Close Config Data.vi"("refnum"=w317) -> ("file path"=w318:path)  [unwired: 2 in, 8 out]
            n211 = call <vilib>:"Open Config Data.vi"("configuration file path"=w318) -> ("refnum"=w316:T11)  [unwired: 8 in, 2 out]
          }
          frame True {
            n212 = property on="Camera Settings" class="Clust (strict)"("Visible"=TRUE) -> ()  [unwired: 2 in, 2 out]
          }
        }
      }
      event "Camera Settings": Value Change {
        n213 = event-data() -> ("NewVal"=w347:T2)  [unwired: 1 in]
        n214 = Index Array(array=w343) -> (element=w342:cluster{string[]})  [unwired: 1 in]
        n215 = Unbundle(w347) -> ("Frame Rate"=w338:i32, "Compression"=w337:i32, "Size"=w340:u16)
        n216 = Unbundle(w342) -> (w341:string[])
        n217 = Index Array(array=w341, index=w340) -> (element=w339:string)
        n218 = Format Into String(format string="%s   %dfps   %d%%", w339, w338, w337) -> (resulting string=w344:string)  [unwired: 2 in, 1 out]
        n219 = Build Array(w344) -> (w345:string[])
        n220 = property on="DB Camera Config" class="Bool (strict)"("Strings [4]"=w345) -> ()  [unwired: 2 in, 2 out]
      }
      event "Motor.Enable": Value Change {
        n221 = event-data() -> ("NewVal"=w353:bool)  [unwired: 1 in]
        n222 = Unbundle("Motor") -> ("Value"=w352:dbl)  [unwired: 1 out]
        n223 = Select(t=w352, s=w353, f=0.0) -> (s? t:f=w350:dbl)
        n224 = call <vilib>:"NT Write Number.vi"("Numeric"=w350, "Name"=w349) -> ()  [unwired: 9 in, 1 out]
      }
      event "Test Slider": Value Change {
        n225 = event-data() -> ("NewVal"=w356:dbl)  [unwired: 1 in]
        n226 = call <vilib>:"NT Write Number.vi"("Numeric"=w356, "Name"=w357) -> ()  [unwired: 9 in, 1 out]
      }
      event "On/Off": Value Change {
        n227 = event-data() -> ("NewVal"=w361:bool)  [unwired: 1 in]
        n228 = Boolean To (0,1)(Boolean=w361) -> (0, 1=w360:i16)
        n229 = call <vilib>:"NT Write Number.vi"("Numeric"=w360, "Name"=w359) -> ()  [unwired: 9 in, 1 out]
      }
      event "Rev/Fwd": Value Change {
        n230 = event-data() -> ("NewVal.Forward"=w369:bool, "NewVal.Reverse"=w368:bool)  [unwired: 1 in]
        n231 = Boolean To (0,1)(Boolean=w369) -> (0, 1=w365:i16)
        n232 = Boolean To (0,1)(Boolean=w368) -> (0, 1=w367:i16)
        n233 = Negate(x=w367) -> (-x=w366:i16)
        n234 = Add(x=w365, y=w366) -> (x+y=w364:i16)
        n235 = call <vilib>:"NT Write Number.vi"("Numeric"=w364, "Name"=w363) -> ()  [unwired: 9 in, 1 out]
      }
      event "Test Ring": Value Change {
        n236 = event-data() -> ("NewVal"=w373:u16)  [unwired: 1 in]
        n237 = property on="Test Ring" class="Ring (strict)"() -> ("Strings []"=w374:string[])  [unwired: 2 in, 2 out]
        n238 = Index Array(array=w374, index=w373) -> (element=w372:string)
        n239 = call <vilib>:"NT Write String.vi"("String"=w372, "Name"=w371) -> ()  [unwired: 9 in, 1 out]
      }
      event "Rec Mode": Value Change {
        # "Update globals for recording mode and path to read log from.\nClear when logging and let NetworkTables set path for vision to\nuse."
        n240 = event-data() -> ("NewVal"=w384:enum32{"Stop", "Record", "Playback"})  [unwired: 1 in]
        n241 = global write "WPI_DashboardLogging Global.vi" "Logging Filename"(path "") -> ()
        n242 = case shown="\"Stop\", \"Record\"" w384 {
          tunnel: w383 -> [_ w386 w394]
          tunnel: [_ _ w393] -> w380
          tunnel: [_ _ w392] -> _
          tunnel: w378 -> [_ _ w390]
          tunnel: cluster{i32, i32} {-250, 170} -> [_ _ w389]
          tunnel: [_ _ T13 {"Image Size"=TRUE, "Image Type"=TRUE, "Pixel Value"=TRUE, "ROI Information"=TRUE, "Zoom Factor"=FALSE} ("Image Information Shown:All Elements")] -> w376
          tunnel: [_ _ TRUE ("Zoom Factor")] -> w375
          frame Default {
          }
          frame "Stop", "Record" {
            # "Place Window too"
            n243 = invoke class="VI" method="FP.Close"(reference=w386) -> (reference out=w385:refnum<vi>)  [unwired: 2 in, 2 out]
            n244 = invoke class="VI" method="Abort VI"(reference=w385) -> ()  [unwired: 2 in, 3 out]
          }
          frame "Playback" {
            n245 = call "Open Playback Panel.vi"("Offset"=w389, "DB VI Ref"=w390, "Playback in"=w394) -> ("Playback out"=w391:refnum<vi>)  [unwired: 8 in]
            n246 = register-events(w391) -> (reference out=w393:refnum<event-registration>, error out=w392:errorcluster)  [unwired: 2 in]
          }
        }
        n247 = global write "WPI_DashboardLogging Global.vi" "Recording"(w384) -> ()
        n248 = property on="Camera Image" class="ImageControl"("Image Information Shown"=w376, "Image Information Visible"=w375) -> ()  [unwired: 2 in, 2 out]
        n249 = call <vilib>:"WPI_DashboardNT Log FieldName Cache.vi"("Operation"=enum16{"Lookup/Add", "Index", "Clear"}."Clear") -> ()  [unwired: 8 in, 3 out]
      }
      event Panel Close {
        w395 = enum32{"Stop", "Record", "Playback"}."Stop" ("Rec Mode")
        n250 = event-data() -> ()  [unwired: 1 in, 4 out]
        n251 = local write "Rec Mode"(w395) -> ()
        n252 = global write "WPI_DashboardLogging Global.vi" "Recording"(w395) -> ()
      }
      event Panel Close {
        # "Abort playback window and ourself"
        n253 = event-data() -> ()  [unwired: 1 in, 4 out]
        n254 = invoke class="VI" method="FP.Close"(reference=w400) -> (reference out=w399:refnum<vi>)  [unwired: 2 in, 2 out]
        n255 = invoke class="VI" method="Abort VI"(reference=w399) -> (error out=w398:errorcluster)  [unwired: 2 in, 2 out]
        n256 = invoke class="VI" method="Abort VI"(error in=w398) -> ()  [unwired: 2 in, 3 out]
      }
    }
  }
  n257 = property on="On/Off" class="Bool (strict)"("Visible"=w25) -> ()  [unwired: 2 in, 2 out]
  n258 = property on="Motor" class="Clust (strict)"("Visible"=w25) -> ()  [unwired: 2 in, 2 out]
  n259 = property on="Progress" class="Clust (strict)"("Visible"=w25) -> ()  [unwired: 2 in, 2 out]
  n260 = property on="Test Ring" class="Ring (strict)"("Visible"=w25) -> ()  [unwired: 2 in, 2 out]
  n261 = property on="Rev/Fwd" class="Clust (strict)"("Visible"=w25) -> ()  [unwired: 2 in, 2 out]
  n262 = property on="Camera Settings" class="Clust (strict)"("Visible"=w25) -> ()  [unwired: 2 in, 2 out]
  n263 = local write "DB Camera Config"(w25) -> ()
  n264 = global write "WPI_DashboardLogging Global.vi" "Recording"(w8) -> ()
  n265 = local write "Rec Mode"(w8) -> ()
